vi "Global 5.vi"() -> ()   [LabVIEW 2014]
uses:
  NavX/roborio/labview/navX-MXP Library/COMMON/TypeDefs/Data TypeDefs/navX Vector Data.ctl
  NavX/roborio/labview/navX-MXP Library/navX-MXP IMU.lvlib
panel:
  in  "IMU_N_Acc":T1
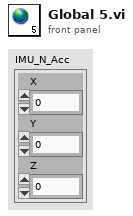
[diagram p1: front panel]
types:
  T1 = typedef "navX-MXP IMU.lvlib/navX Vector Data.ctl" = cluster{"X":dbl, "Y":dbl, "Z":dbl}
diagram:
